vi "Navigation_Main_position_testing april 19.vi"() -> ()   [LabVIEW 2015]
uses:
  <vilib>/myRIO/Common/Instrument Driver Framework/Utilities/typedefs/Generic FPGA Reference.ctl
  <vilib>/myRIO/Common/Instrument Driver Framework/Utilities/typedefs/myRIO v1.0 Reference.ctl
  <vilib>/myRIO/Common/Instrument Driver Framework/Utilities/typedefs/Hardware Version Enum.ctl
  <vilib>/myRIO/Common/Instrument Driver Framework/Utilities/typedefs/myRIO Generic Hardware Reference.ctl
  <vilib>/userdefined/High Color/nirio_resource_hc.ctl
  <vilib>/myRIO/Instrument Drivers/Onboard IO/PWM/typedefs/PWM Configuration.ctl
  <vilib>/myRIO/Instrument Drivers/Onboard IO/PWM/PWM.lvlib
  <vilib>/myRIO/Common/Instrument Driver Framework/myRIO v1.0/PWM/typedefs/PWM Channels Enum.ctl
  <vilib>/myRIO/Instrument Drivers/Onboard IO/PWM/typedefs/PWM Reference.ctl
  <vilib>/myRIO/Instrument Drivers/Onboard IO/PWM/vis/myRIO PWM Open.xnode
  <vilib>/myRIO/Common/Instrument Driver Framework/myRIO v1.0/PWM/vis/myRIO v1.1 Open PWM.vi
  <vilib>/rvi/interface/nirviOpenFPGA/nirviOpenFPGA.xnode
  <vilib>/myRIO/Instrument Drivers/Utilities/Utilities.lvlib
  <vilib>/rvi/interface/nirviReadWriteControl/nirviReadWriteControl.xnode
  NiFpgaLv.dll
  <vilib>/Utility/error.llb/Error Cluster From Error Code.vi
  <vilib>/rvi/interface/Simulation/niFpgaSimulationCallBeginRW.vi
  <vilib>/rvi/errors/niLvFpgaAdjustHostInterfaceError.vi
  Navi/E/FPGA Bitfiles/NavigationProjec_FPGATarget2_FPGAMainNavigati_PWPHW8gwDxI.lvbitx
  <vilib>/addons/control/pid/NI_PID_pid.lvlib
  <vilib>/addons/control/pid/pid.llb/PID (DBL).vi
  <vilib>/FPGAPlugInAG/myRIO-1900/niLvFpga_Open_myRIO-1900.vi
  <vilib>/rvi/interface/common/dynamic/niFpgaDynamicAddResources.vi
panel:
  in  "Boolean":bool=TRUE
  out "stop switch":dbl=1.0
  out "distance to goal":dbl
  out "loc_y":dbl
  out "loc_x":dbl
  out "loc_theta":dbl
  out "start y":dbl
  out "start angle":dbl=1.0
  out "start x":dbl=1.0
  in  "set start position":bool=TRUE
  out "goal reached":bool=TRUE
  out "x/y":dbl
  out "scale":dbl=1.0
  in  "x goal":dbl=10.0
  in  "L Desired Input Velocity (ft/s) 4":dbl(knob) scale=-4.0..4.0
  in  "R Min Linear Velocity (ft/s)  2":dbl=-2.0 format="%#_13g"
  in  "L Min Linear Velocity (ft/s) 9":dbl=-2.0 format="%#_13g"
  in  "R Max Linear Velocity (ft/s) 5":dbl=2.0 format="%#_13g"
  in  "L Max Linear Velocity (ft/s) 5":dbl=2.0 format="%#_13g"
  in  "R Desired Input Velocity (ft/s) 5":dbl(knob) scale=-4.0..4.0
  out "left":dbl
  out "right":dbl
  out "left wheels actual pwm":dbl
  in  "stop 3":bool
  out "left pwm":dbl(graph)
  out "dt out (s) 3":dbl format="%.3f"
  in  "output range 3":cluster{"output high":dbl, "output low":dbl}={"output high"=0.13333, "output low"=-0.13333} {"output low" format="%.6f"; "output high" format="%.5f"}
  in  "PID gains 3":T1={"proportional gain (Kc)"=0.002, "integral time (Ti, min)"=7e-07, "derivative time (Td, min)"=0.0} {"derivative time (Td, min)" format="%.8f"; "integral time (Ti, min)" format="%.8f"; "proportional gain (Kc)" format="%.8f"}
  out "desired pwm 2":dbl
  out "feedback 2":dbl
  out ".not. x? 3":bool
  out "Elapsed Time (s) 2":dbl caption="Elapsed Time (s)"
  out "x traveled 2":dbl
  out "y traveled 2":dbl
  out "avg 124":dbl
  out "avg 457":dbl
  out "psi dot 2":dbl
  out "distance traveled 2":dbl
  out "y dot 2":dbl
  out "x dot 2":dbl
  out "x position 2":dbl
  out "y position 2":dbl
  out "reset x y 2":dbl
  out "Tick Count(mSec) 2":u32 caption="Tick Count(mSec)"
  in  "start y 2":dbl=3.0
  in  "start x 2":dbl=1.0
  out "right wheels actual pwm":dbl
  in  "stop 2":bool
  out "right pwm":dbl(graph)
  out "dt out (s) 2":dbl format="%.3f"
  in  "output range 2":cluster{"output high":dbl, "output low":dbl}={"output high"=0.13333, "output low"=-0.13333} {"output low" format="%.6f"; "output high" format="%.5f"}
  in  "PID gains 2":T1={"proportional gain (Kc)"=0.002, "integral time (Ti, min)"=7e-07, "derivative time (Td, min)"=0.0} {"derivative time (Td, min)" format="%.8f"; "integral time (Ti, min)" format="%.8f"; "proportional gain (Kc)" format="%.8f"}
  out "desired pwm":dbl
  out "feedback":dbl
  out ".not. x? 2":bool
  out "Elapsed Time (s)":dbl
  out "LF Rot Velocity (rot/s)":dbl
  out "LM Rot Velocity (rot/s)":dbl
  out "LR Rot Velocity (rot/s)":dbl
  out "RR Rot Velocity (rot/s)":dbl
  out "RM Linear Velocity (rot/s)":dbl
  out "RF Linear Velocity (rot/s)":dbl
  in  "Encoder Reset":bool
  out "SYS.SELECTA":u8 format="%08b"
  out "ENC.B_c.CNTR":i32
  out "ENC.B_b.CNTR":i32
  out "ENC.B_a.CNTR":i32
  out "ENC.A_c.CNTR":i32
  out "ENC.A_b.CNTR":i32
  out "ENC.A_a.CNTR":i32
  in  "R Min Linear Velocity (ft/s)":dbl=-2.0 format="%#_13g"
  in  "R Max Linear Velocity (ft/s)":dbl=2.0 format="%#_13g"
  in  "L Min Linear Velocity (ft/s)":dbl=-2.0 format="%#_13g"
  in  "L Max Linear Velocity (ft/s)":dbl=2.0 format="%#_13g"
  out "Current Rot Velocity (rot/s)":T2(graph)
  # "Motor Control Parameters"
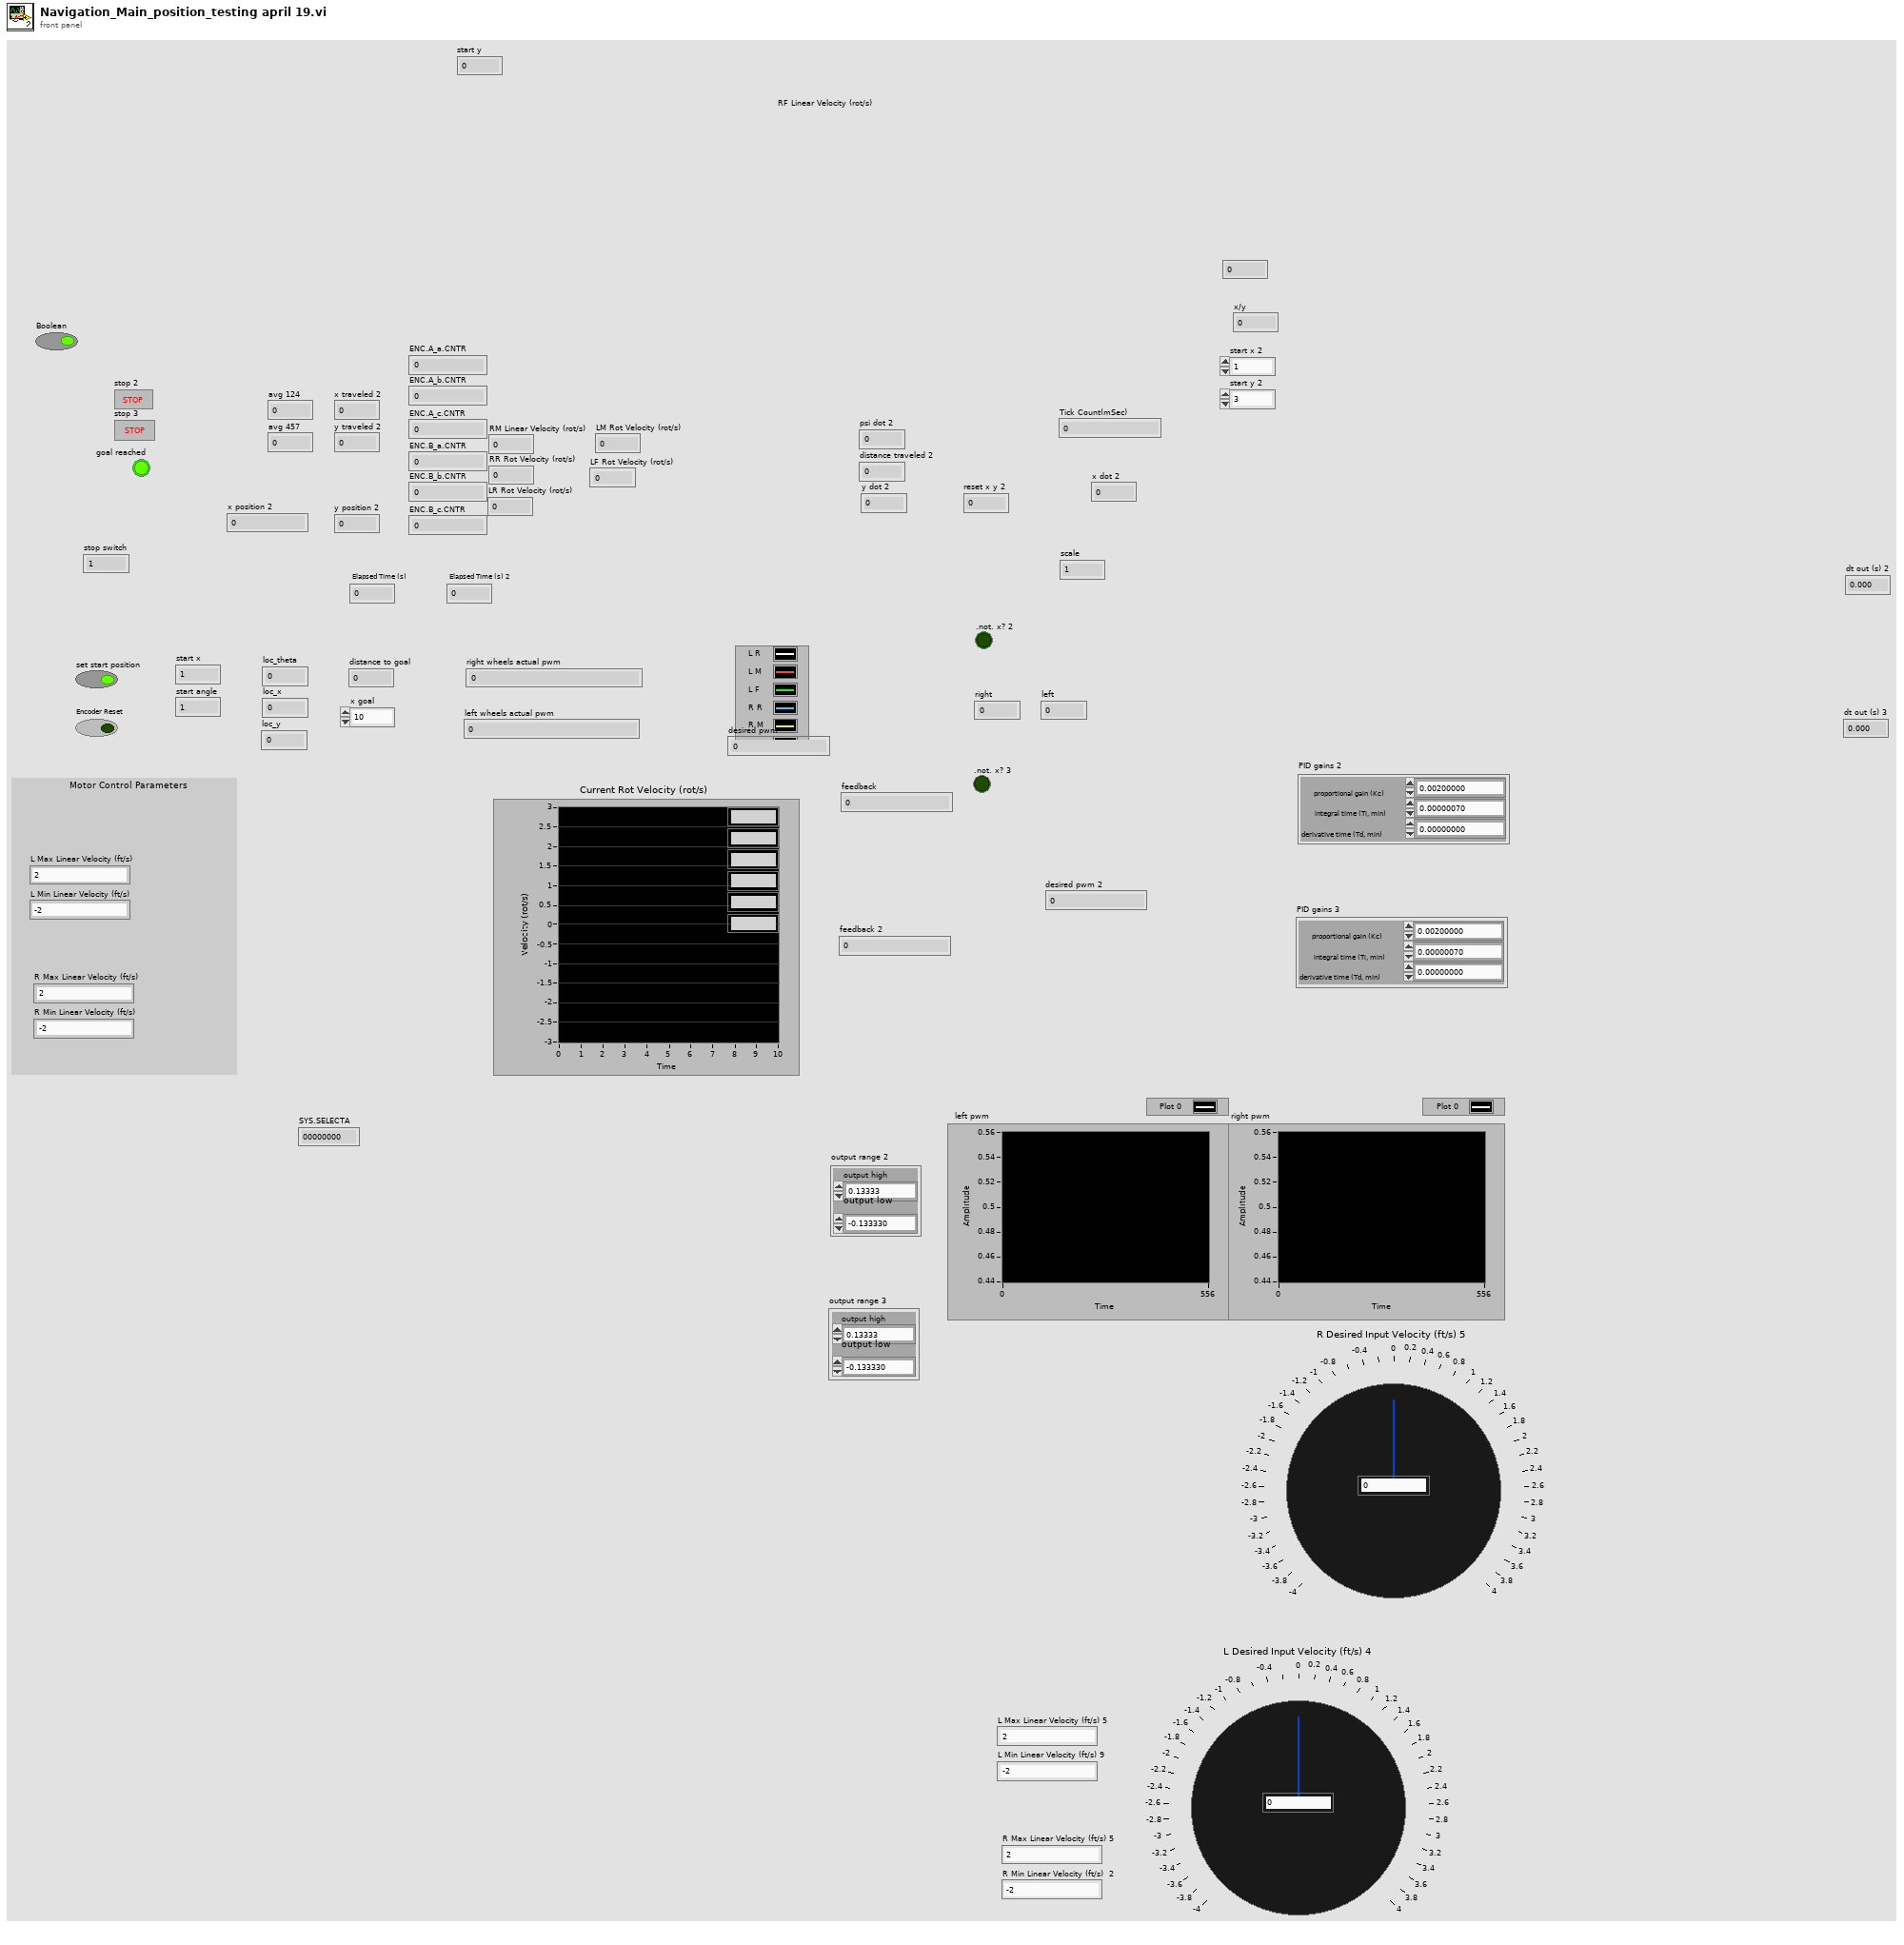
[diagram p1: front panel]
types:
  T1 = cluster{"proportional gain (Kc)":dbl, "integral time (Ti, min)":dbl, "derivative time (Td, min)":dbl}
  T2 = cluster{"Rotational Velocity (RPS)":dbl, "Rotational Velocity (RPS)":dbl, "Rotational Velocity (RPS)":dbl, "Rotational Velocity (RPS)":dbl, "Rotational Velocity (RPS)":dbl, "Rotational Velocity (RPS)":dbl}
  T3 = typedef "nirio_resource_hc.ctl" = tag
  T4 = typedef "Hardware Version Enum.ctl" = enum16{"Unknown", "myRIO-1900", "myRIO-1950", "roboRIO"}
  T5 = typedef "PWM.lvlib/PWM Reference.ctl" = cluster{"myRIO Reference":T6, "PWM Channels Enum":T9, "PWM Configuration":T10}
  T6 = typedef "myRIO Generic Hardware Reference.ctl" = cluster{"myRIO Model":T4, "myRIO Hardware Reference":T7}
  T7 = typedef "myRIO v1.0 Reference.ctl" = cluster{"Generic FPGA Reference":T8, "Allow multiple opens":bool}
  T8 = typedef "Generic FPGA Reference.ctl" = refnum<k20>
  T9 = typedef "PWM Channels Enum.ctl" = enum16{"Not Connected", "C/PWM0", "C/PWM1", "A/PWM0", "A/PWM1", "A/PWM2", "B/PWM0", "B/PWM1", "B/PWM2", "PWM/PWM0", "PWM/PWM1", "PWM/PWM2", "PWM/PWM3", "PWM/PWM4", "PWM/PWM5", "PWM/PWM6", "PWM/PWM7", "PWM/PWM8", "PWM/PWM9"}
  T10 = typedef "PWM.lvlib/PWM Configuration.ctl" = cluster{"Frequency":dbl, "Duty Cycle":dbl}
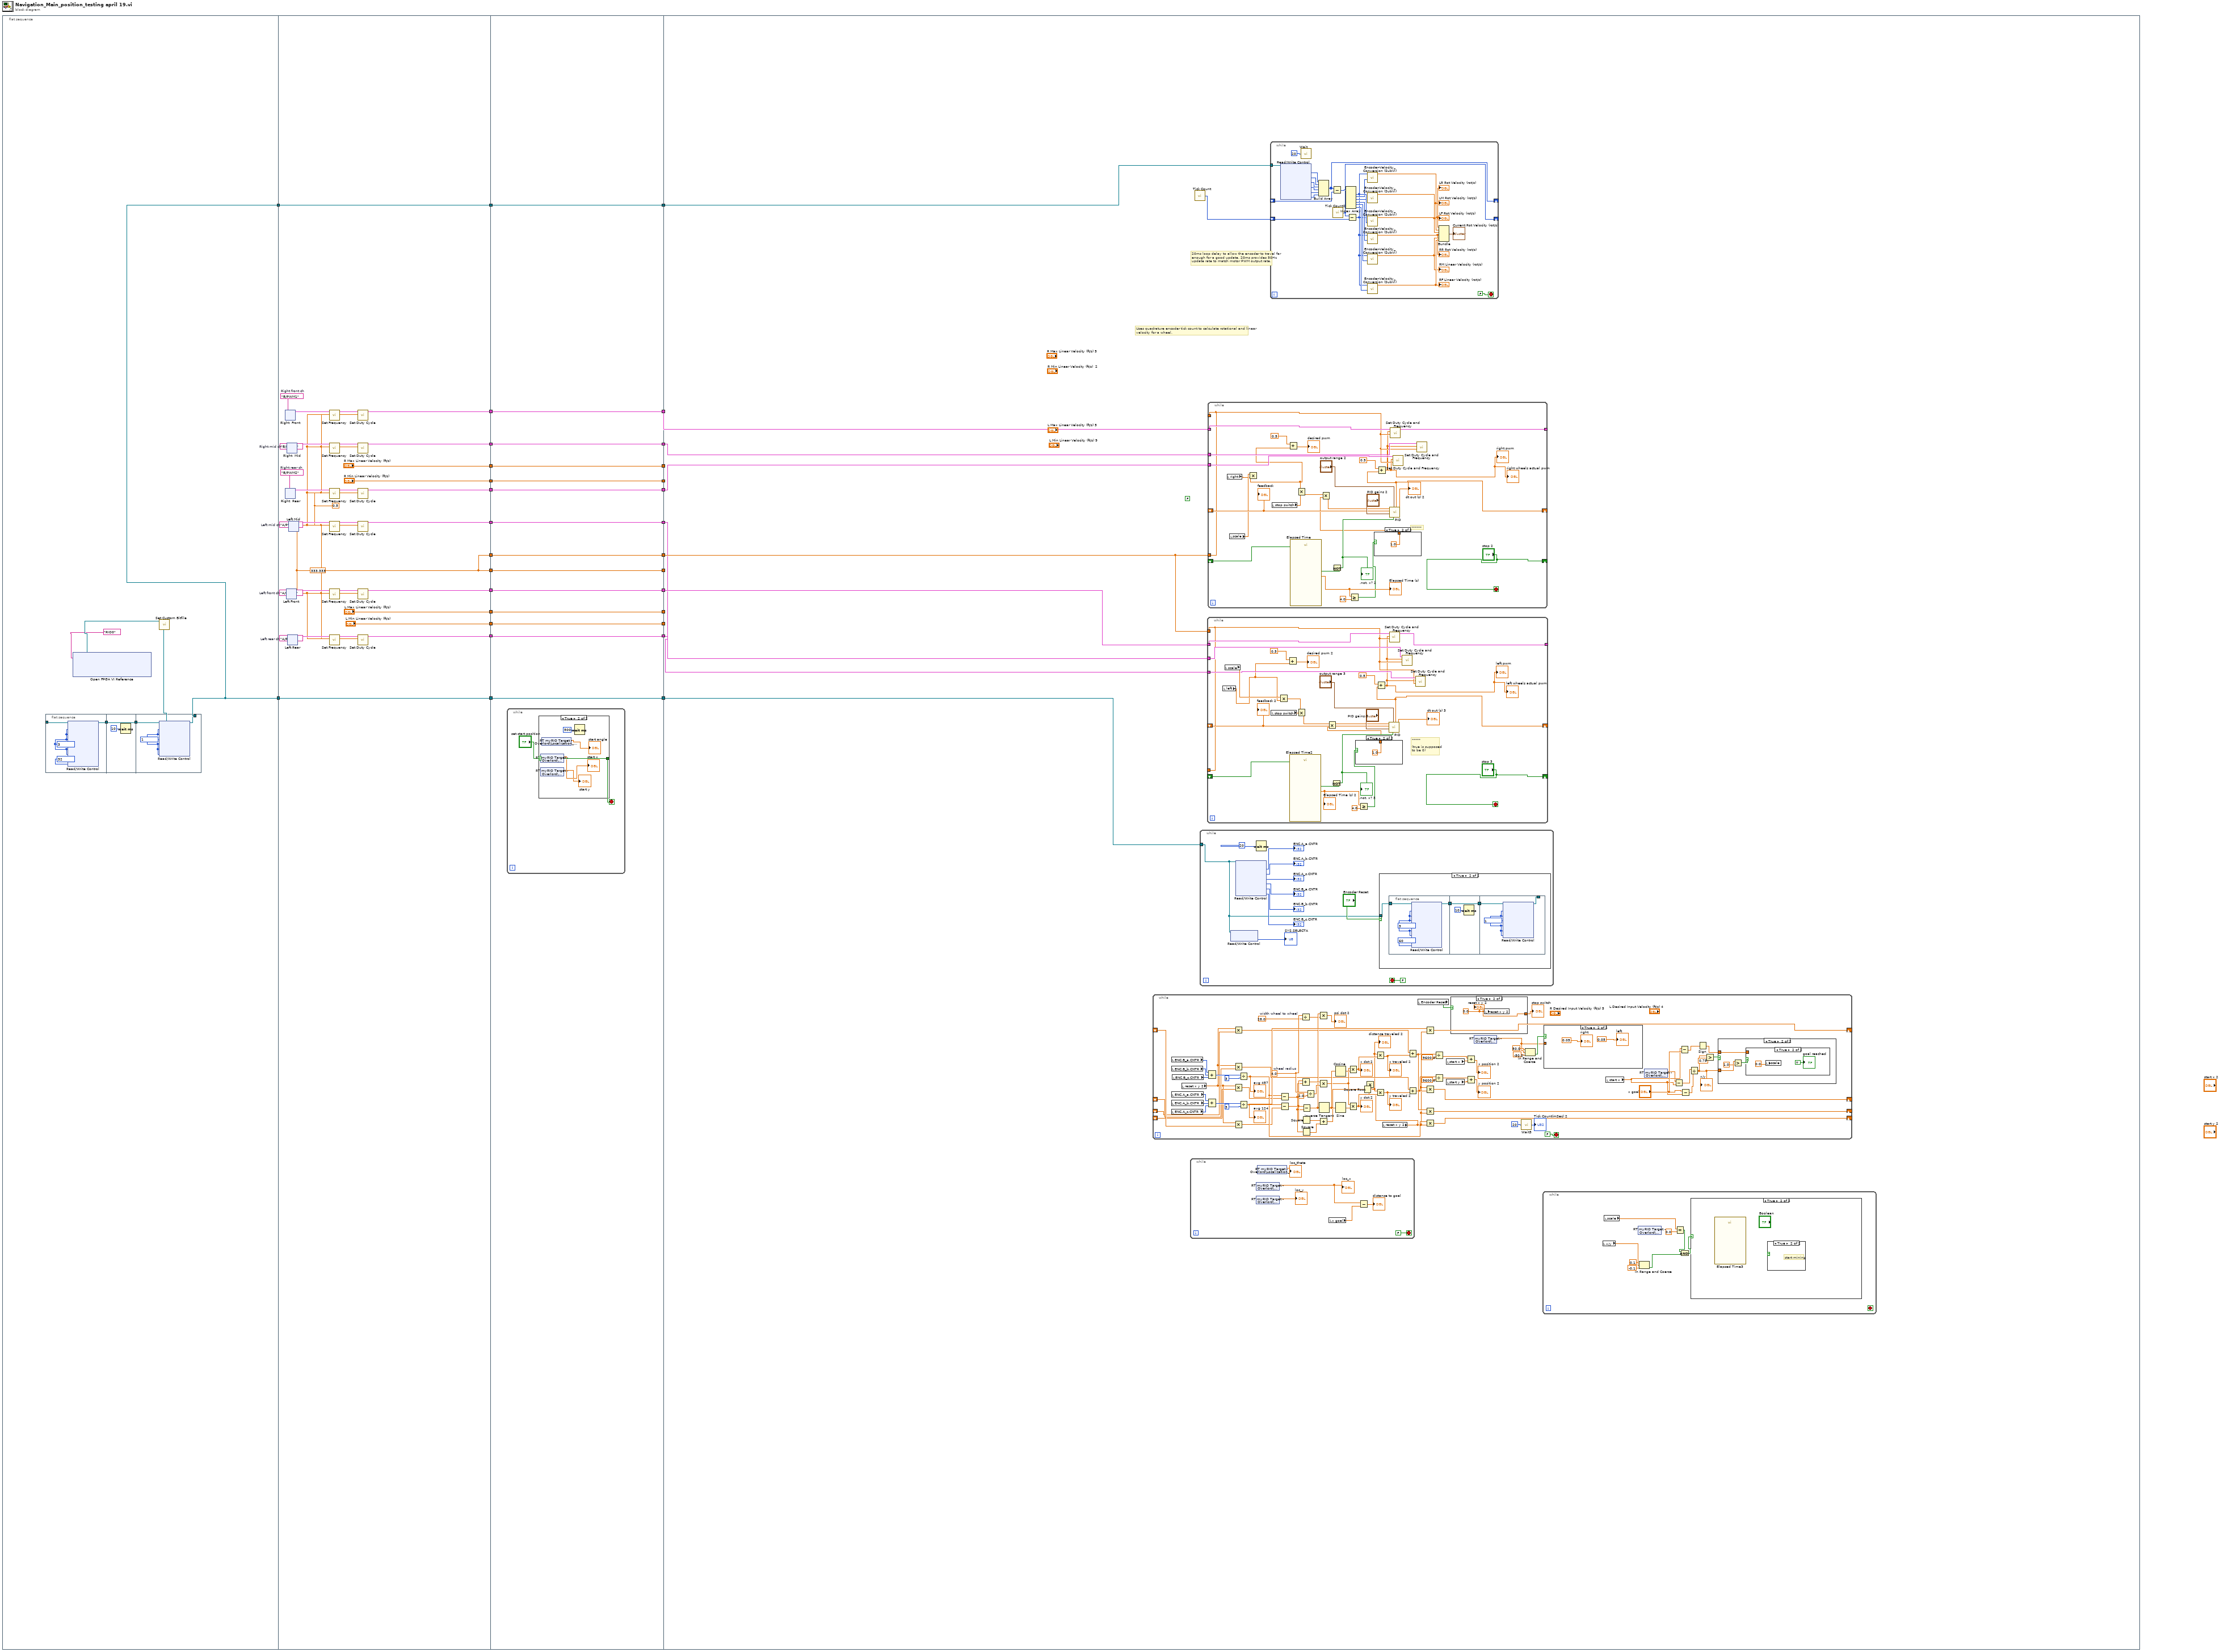
[diagram p0: block diagram]
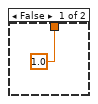
[diagram p5: hidden frame]
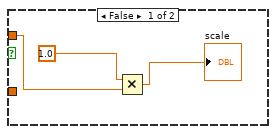
[diagram p6: hidden frame]
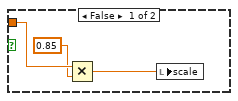
[diagram p7: hidden frame]
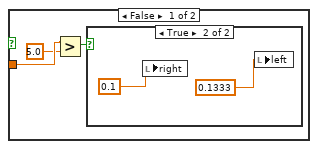
[diagram p8: hidden frame]
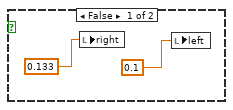
[diagram p9: hidden frame]
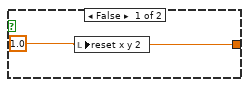
[diagram p10: hidden frame]
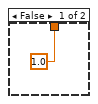
[diagram p11: hidden frame]
diagram:
  n1 = flat-sequence {
    tunnel: [w33] -> w30
    tunnel: [w33] -> w29
    tunnel: [w46] -> w28
    tunnel: [w61] -> w26
    tunnel: [w57] -> w24
    tunnel: [w56] -> w22
    tunnel: [w55] -> w20
    tunnel: [w54] -> w18
    tunnel: [w53] -> w16
    tunnel: ["L Max Linear Velocity (ft/s)"] -> w14
    tunnel: ["L Min Linear Velocity (ft/s)"] -> w12
    tunnel: ["R Max Linear Velocity (ft/s)"] -> w10
    tunnel: ["R Min Linear Velocity (ft/s)"] -> w8
    tunnel: [w48] -> w6
    tunnel: w30 -> [w47]
    tunnel: [w47] -> w4
    tunnel: w29 -> [w48]
    tunnel: [w46] -> w2
    tunnel: w28 -> [w187]
    tunnel: [w187] -> w27
    tunnel: w26 -> [w186]
    tunnel: [w186] -> w25
    tunnel: w24 -> [w185]
    tunnel: [w185] -> w23
    tunnel: w22 -> [w184]
    tunnel: [w184] -> w21
    tunnel: w20 -> [w183]
    tunnel: [w183] -> w19
    tunnel: w18 -> [w182]
    tunnel: [w182] -> w17
    tunnel: w16 -> [w181]
    tunnel: [w181] -> w15
    tunnel: w14 -> [w180]
    tunnel: [w180] -> w13
    tunnel: w12 -> [w179]
    tunnel: [w179] -> w11
    tunnel: w10 -> [w178]
    tunnel: [w178] -> w9
    tunnel: w8 -> [w177]
    tunnel: [w177] -> w7
    tunnel: w6 -> [w176]
    tunnel: [w176] -> w5
    tunnel: w4 -> [w175]
    tunnel: [w175] -> w3
    tunnel: w2 -> [w174]
    tunnel: [w174] -> w1
    tunnel: w27 -> [_]
    tunnel: w25 -> [w195]
    tunnel: w23 -> [w201]
    tunnel: w21 -> [w198]
    tunnel: w19 -> [w197]
    tunnel: w17 -> [w196]
    tunnel: w15 -> [w200]
    tunnel: w13 -> [_]
    tunnel: w11 -> [_]
    tunnel: w9 -> [_]
    tunnel: w7 -> [_]
    tunnel: w5 -> [w203]
    tunnel: w3 -> [w202]
    tunnel: w1 -> [w199]
    frame #0 {
      n2 = flat-sequence {
        tunnel: w34 -> [w39]
        tunnel: [w37] -> w36
        tunnel: w36 -> [w41]
        tunnel: [w41] -> w35
        tunnel: w35 -> [w44]
        tunnel: [w43] -> w33
        frame #0 {
          w38 = u8 32 ("SYS.SELECTA")
          w40 = u8 3 ("ENC.B_c.CNFG")
          n3 = xnode "Read/Write Control"("FPGA VI Reference In"=w39, "ENC.A_a.CNFG"=w40, "ENC.A_b.CNFG"=w40, "ENC.A_c.CNFG"=w40, "ENC.B_a.CNFG"=w40, "ENC.B_b.CNFG"=w40, "ENC.B_c.CNFG"=w40, "SYS.SELECTA"=w38, "SYS.SELECTB"=w38) -> ("FPGA VI Reference Out"=w37:refnum<k20>)  [unwired: 1 in, 1 out]
        }
        frame #1 {
          n4 = Wait (ms)(milliseconds to wait=u32 10) -> ()  [unwired: 1 out]
        }
        frame #2 {
          w45 = u8 1 ("ENC.B_c.CNFG")
          n5 = xnode "Read/Write Control"("FPGA VI Reference In"=w44, "ENC.A_a.CNFG"=w45, "ENC.A_b.CNFG"=w45, "ENC.A_c.CNFG"=w45, "ENC.B_a.CNFG"=w45, "ENC.B_b.CNFG"=w45, "ENC.B_c.CNFG"=w45) -> ("FPGA VI Reference Out"=w43:refnum<k20>)  [unwired: 1 in, 1 out]
        }
      }
      n6 = xnode "Open FPGA VI Reference"("resource name"=tag "RIO0") -> ("FPGA VI Reference Out"=w32:refnum<k20>)  [unwired: 1 in, 1 out]
      n7 = call <vilib>:"Set Custom Bitfile.vi"("Custom FPGA Reference In"=w32) -> ("Custom FPGA Reference Out"=w34:refnum<k20>)  [unwired: 9 in, 1 out]
    }
    frame #1 {
      w58 = 0.5 ("Duty Cycle")
      w46 = 333.333 ("Frequency [Hz]")
      w72 = tag "B/PWM2"  # Right rear ch
      w73 = tag "B/PWM0"  # Right mid ch
      w74 = tag "B/PWM1"  # Right front ch
      w75 = tag "A/PWM2"  # Left rear ch
      w76 = tag "A/PWM1"  # Left mid ch
      w77 = tag "A/PWM0"  # Left front ch
      n8 = xnode "Right  Front"("Channel Name"=w74) -> ("PWM Ref Out"=w68:T5)  [unwired: 2 in, 1 out]
      n9 = xnode "Right  Rear"("Channel Name"=w72) -> ("PWM Ref Out"=w66:T5)  [unwired: 2 in, 1 out]
      n10 = xnode "Left Front"("Channel Name"=w77) -> ("PWM Ref Out"=w71:T5)  [unwired: 2 in, 1 out]
      n11 = xnode "Right  Mid"("Channel Name"=w73) -> ("PWM Ref Out"=w67:T5)  [unwired: 2 in, 1 out]
      n12 = xnode "Left Rear"("Channel Name"=w75) -> ("PWM Ref Out"=w69:T5)  [unwired: 2 in, 1 out]
      n13 = xnode "Left Mid"("Channel Name"=w76) -> ("PWM Ref Out"=w70:T5)  [unwired: 2 in, 1 out]
      n14 = call <vilib>:"Set Frequency.vi"("Frequency [Hz]"=w46, "PWM Ref In"=w68) -> ("PWM Ref Out"=w62:T5)  [unwired: 7 in, 1 out]
      n15 = call <vilib>:"Set Frequency.vi"("Frequency [Hz]"=w46, "PWM Ref In"=w67) -> ("PWM Ref Out"=w63:T5)  [unwired: 7 in, 1 out]
      n16 = call <vilib>:"Set Frequency.vi"("Frequency [Hz]"=w46, "PWM Ref In"=w66) -> ("PWM Ref Out"=w64:T5)  [unwired: 7 in, 1 out]
      n17 = call <vilib>:"Set Frequency.vi"("Frequency [Hz]"=w46, "PWM Ref In"=w70) -> ("PWM Ref Out"=w59:T5)  [unwired: 7 in, 1 out]
      n18 = call <vilib>:"Set Frequency.vi"("Frequency [Hz]"=w46, "PWM Ref In"=w71) -> ("PWM Ref Out"=w65:T5)  [unwired: 7 in, 1 out]
      n19 = call <vilib>:"Set Frequency.vi"("Frequency [Hz]"=w46, "PWM Ref In"=w69) -> ("PWM Ref Out"=w60:T5)  [unwired: 7 in, 1 out]
      n20 = call <vilib>:"Set Duty Cycle.vi"("Duty Cycle"=w58, "PWM Ref In"=w62) -> ("PWM Ref Out"=w57:T5)  [unwired: 7 in, 1 out]
      n21 = call <vilib>:"Set Duty Cycle.vi"("Duty Cycle"=w58, "PWM Ref In"=w63) -> ("PWM Ref Out"=w56:T5)  [unwired: 7 in, 1 out]
      n22 = call <vilib>:"Set Duty Cycle.vi"("Duty Cycle"=w58, "PWM Ref In"=w64) -> ("PWM Ref Out"=w55:T5)  [unwired: 7 in, 1 out]
      n23 = call <vilib>:"Set Duty Cycle.vi"("Duty Cycle"=w58, "PWM Ref In"=w59) -> ("PWM Ref Out"=w54:T5)  [unwired: 7 in, 1 out]
      n24 = call <vilib>:"Set Duty Cycle.vi"("Duty Cycle"=w58, "PWM Ref In"=w65) -> ("PWM Ref Out"=w53:T5)  [unwired: 7 in, 1 out]
      n25 = call <vilib>:"Set Duty Cycle.vi"("Duty Cycle"=w58, "PWM Ref In"=w60) -> ("PWM Ref Out"=w61:T5)  [unwired: 7 in, 1 out]
    }
    frame #2 {
      n26 = while {
        stop <- w188 stop-if-true
        n27 = case shown="True" "set start position" {
          selector: "set start position" -> [_ w194]
          tunnel: [_ w194] -> w188
          frame False {
          }
          frame True {
            n28 = shared-variable "RT myRIO Target - Overlord\\Localization_Variables_r0.lvlib\\loc_x"() -> (→"start x":dbl)  [unwired: 1 in, 1 out]
            n29 = shared-variable "RT myRIO Target - Overlord\\Localization_Variables_r0.lvlib\\loc_y"() -> (→"start y":dbl)  [unwired: 1 in, 1 out]
            n30 = shared-variable "RT myRIO Target - Overlord\\Localization_Variables_r0.lvlib\\loc_theta"() -> (→"start angle":dbl)  [unwired: 1 in, 1 out]
            n31 = Wait (ms)(milliseconds to wait=u32 500) -> ()  [unwired: 1 out]
          }
        }
      }
    }
    frame #3 {
      (unwired) FALSE
      # "Uses quadrature encoder tick count to calculate rotational and linear velocity for a wheel."
      # "20ms loop delay to allow the encoder to travel far enough for a good update. 20ms provides 50Hz update rate to match motor PWM output rate."
      n32 = while {
        shift-right: [w275] -> _
        shift-left: _ -> [w313]
        shift-right: [w272] -> _
        shift-left: _ -> [w312]
        shift-right: [w274] -> _
        shift-left: _ -> [w287]
        shift-right: [w273] -> _
        shift-left: _ -> [w286]
        stop <- FALSE stop-if-true
        w308 = 28.0  # width wheel to wheel
        w309 = 4.0  # wheel radius
        n33 = local read "ENC.B_a.CNTR"() -> (w318:i32)
        n34 = local read "ENC.B_b.CNTR"() -> (w317:i32)
        n35 = local read "ENC.A_a.CNTR"() -> (w321:i32)
        n36 = local read "ENC.A_b.CNTR"() -> (w320:i32)
        n37 = local read "ENC.A_c.CNTR"() -> (w319:i32)
        n38 = local read "ENC.B_c.CNTR"() -> (w316:i32)
        n39 = local read "reset x y 2"() -> (w271:dbl)
        n40 = Compound Arithmetic op=ADD(w318, w317, w316) -> (w324:i32)
        n41 = Compound Arithmetic op=ADD(w321, w320, w319) -> (w325:i32)
        n42 = Multiply(x=w271, y=w286) -> (x*y=w277:dbl)
        n43 = Multiply(x=w271, y=w287) -> (x*y=w278:dbl)
        n44 = Multiply(x=w271, y=w312) -> (x*y=w276:dbl)
        n45 = Multiply(x=w271, y=w313) -> (x*y=w279:dbl)
        n46 = Divide(x=w324, y=3) -> (x/y=w311:dbl)
        "avg 457" <- w311
        n47 = Divide(x=w325, y=3) -> (x/y=w314:dbl)
        "avg 124" <- w314
        n48 = Subtract(x=w311, y=w276) -> (x-y=w301:dbl)
        n49 = Subtract(x=w314, y=w279) -> (x-y=w302:dbl)
        n50 = Divide(x=w309, y=w308) -> (x/y=w304:dbl)
        n51 = Add(x=w302, y=w301) -> (x+y=w306:dbl)
        n52 = Square(x=w302) -> (x^2=w299:dbl)
        n53 = Square(x=w301) -> (x^2=w300:dbl)
        n54 = Subtract(x=w302, y=w301) -> (x-y=w305:dbl)
        n55 = Divide(x=w309, y=2.0) -> (x/y=w307:dbl)
        n56 = Multiply(x=w305, y=w304) -> (x*y=→"psi dot 2":dbl)
        n57 = Multiply(x=w306, y=w307) -> (x*y=w295:dbl)
        n58 = Add(x=w299, y=w300) -> (x+y=w298:dbl)
        n59 = Inverse Tangent(1:w305) -> (0:w303:dbl)
        n60 = Cosine(x=w303) -> (cos(x)=w296:dbl)
        n61 = Sine(x=w303) -> (sin(x)=w297:dbl)
        n62 = Multiply(x=w295, y=w296) -> (x*y=w293:dbl)
        "x dot 2" <- w293
        n63 = Multiply(x=w295, y=w297) -> (x*y=w294:dbl)
        "y dot 2" <- w294
        n64 = Square Root(x=w298) -> (sqrt(x)=w292:dbl)
        n65 = local read "reset x y 2"() -> (w269:dbl)
        n66 = Multiply(x=w292, y=w269) -> (x*y=w270:dbl)
        "distance traveled 2" <- w270
        n67 = Multiply(x=w270, y=w293) -> (x*y=w291:dbl)
        "x traveled 2" <- w291
        n68 = Multiply(x=w270, y=w294) -> (x*y=w290:dbl)
        "y traveled 2" <- w290
        n69 = Add(x=w277, y=w291) -> (x+y=w289:dbl)
        n70 = Add(x=w278, y=w290) -> (x+y=w281:dbl)
        n71 = local read "Encoder Reset"() -> (w268:bool)
        n72 = Multiply(x=w314, y=w269) -> (x*y=w275:dbl)
        n73 = Multiply(x=w269, y=w281) -> (x*y=w274:dbl)
        n74 = Multiply(x=w289, y=w269) -> (x*y=w273:dbl)
        n75 = Multiply(x=w311, y=w269) -> (x*y=w272:dbl)
        n76 = Divide(x=w289, y=9600.0) -> (x/y=w284:dbl)
        n77 = Divide(x=w281, y=9600.0) -> (x/y=w285:dbl)
        n78 = local read "start x"() -> (w282:dbl)
        n79 = local read "start y"() -> (w283:dbl)
        n80 = case shown="True" w268 {
          tunnel: [w348 w349] -> w249
          frame False {
            w348 = 1.0
            n81 = local write "reset x y 2"(w348) -> ()
          }
          frame True {
            w349 = 0.0
            n82 = local write "reset x y 2"(w349) -> ()
            "reset x y 2" <- w349
          }
        }
        "stop switch" <- w249
        n83 = Add(x=w284, y=w282) -> (x+y=→"x position 2":dbl)
        n84 = Add(x=w285, y=w283) -> (x+y=→"y position 2":dbl)
        n85 = shared-variable "RT myRIO Target - Overlord\\Localization_Variables_r0.lvlib\\loc_x"() -> (w251:dbl)  [unwired: 1 in, 1 out]
        n86 = call "Wait3"("Count(mSec)"=u32 20) -> ("Tick Count(mSec)"=→"Tick Count(mSec) 2":u32)
        n87 = In Range and Coerce(upper limit=50.0, x=w251, lower limit=-50.0) -> (In Range?=w262:bool)  [unwired: 1 out]
        n88 = case shown="True" w262 {
          tunnel: w251 -> [w341 _]
          frame False {
            n89 = Greater?(x=w341, y=5.0) -> (0:w339:bool)
            n90 = case shown="True" w339 {
              frame False {
                n91 = local write "right"(0.133) -> ()
                n92 = local write "left"(0.1) -> ()
              }
              frame True {
                n93 = local write "right"(0.1) -> ()
                n94 = local write "left"(0.1333) -> ()
              }
            }
          }
          frame True {
            "right" <- 0.05
            "left" <- 0.05
          }
        }
        n95 = local read "start x"() -> (w253:dbl)
        n96 = shared-variable "RT myRIO Target - Overlord\\Localization_Variables_r0.lvlib\\loc_x"() -> (w250:dbl)  [unwired: 1 in, 1 out]
        n97 = Subtract(x=w250, y=w253) -> (x-y=w258:dbl)
        n98 = Subtract(x=w253, y="x goal") -> (x-y=w255:dbl)
        n99 = Subtract(x="x goal", y=w253) -> (x-y=w257:dbl)
        n100 = Divide(x=w258, y=w257) -> (x/y=w259:dbl)
        "x/y" <- w259
        n101 = Sign(1:w255) -> (0:w254:dbl)
        n102 = Greater?(x=w259, y=0.75) -> (0:w260:bool)
        n103 = case shown="True" w260 {
          tunnel: w259 -> [_ w333]
          tunnel: w254 -> [w328 w330]
          frame False {
            n104 = Multiply(x=1.0, y=w328) -> (x*y=→"scale":dbl)
          }
          frame True {
            n105 = Greater?(x=w333, y=1.0) -> (0:w331:bool)
            n106 = case shown="True" w331 {
              tunnel: w330 -> [w336 _]
              frame False {
                n107 = Multiply(x=w336, y=0.85) -> (x*y=w334:dbl)
                n108 = local write "scale"(w334) -> ()
              }
              frame True {
                n109 = local write "scale"(0.0) -> ()
                "goal reached" <- TRUE
              }
            }
          }
        }
      }
      n110 = while {
        stop <- FALSE stop-if-true
        n111 = shared-variable "RT myRIO Target - Overlord\\Localization_Variables_r0.lvlib\\loc_x"() -> (w216:dbl)  [unwired: 1 in, 1 out]
        "loc_x" <- w216
        n112 = shared-variable "RT myRIO Target - Overlord\\Localization_Variables_r0.lvlib\\loc_y"() -> (→"loc_y":dbl)  [unwired: 1 in, 1 out]
        n113 = shared-variable "RT myRIO Target - Overlord\\Localization_Variables_r0.lvlib\\loc_theta"() -> (→"loc_theta":dbl)  [unwired: 1 in, 1 out]
        n114 = local read "x goal"() -> (w215:dbl)
        n115 = Subtract(x=w216, y=w215) -> (x-y=→"distance to goal":dbl)
      }
      n116 = call "Tick Count"() -> ("Tick Count(uSec)"=w204:u32)
      n117 = while {
        tunnel: w203 -> [w380]
        stop <- FALSE stop-if-true
        n118 = xnode "Read/Write Control"("FPGA VI Reference In"=w380) -> ("SYS.SELECTA"=→"SYS.SELECTA":u8)  [unwired: 1 in, 2 out]
        n119 = xnode "Read/Write Control"("FPGA VI Reference In"=w380) -> ("ENC.A_a.CNTR"=→"ENC.A_a.CNTR":u32, "ENC.A_b.CNTR"=→"ENC.A_b.CNTR":u32, "ENC.A_c.CNTR"=→"ENC.A_c.CNTR":u32, "ENC.B_a.CNTR"=→"ENC.B_a.CNTR":u32, "ENC.B_b.CNTR"=→"ENC.B_b.CNTR":u32, "ENC.B_c.CNTR"=→"ENC.B_c.CNTR":u32)  [unwired: 1 in, 2 out]
        n120 = Wait (ms)(milliseconds to wait=u32 20) -> ()  [unwired: 1 out]
        n121 = case shown="True" "Encoder Reset" {
          tunnel: w380 -> [_ w391]
          frame False {
          }
          frame True {
            n122 = flat-sequence {
              tunnel: w391 -> [w396]
              tunnel: [w394] -> w393
              tunnel: w393 -> [w398]
              tunnel: [w398] -> w392
              tunnel: w392 -> [w401]
              tunnel: [w400] -> _
              frame #0 {
                w395 = u8 60 ("SYS.SELECTA")
                w397 = u8 3 ("ENC.B_c.CNFG")
                n123 = xnode "Read/Write Control"("FPGA VI Reference In"=w396, "ENC.A_a.CNFG"=w397, "ENC.A_b.CNFG"=w397, "ENC.A_c.CNFG"=w397, "ENC.B_a.CNFG"=w397, "ENC.B_b.CNFG"=w397, "ENC.B_c.CNFG"=w397, "SYS.SELECTA"=w395, "SYS.SELECTB"=w395) -> ("FPGA VI Reference Out"=w394:refnum<k20>)  [unwired: 1 in, 1 out]
              }
              frame #1 {
                n124 = Wait (ms)(milliseconds to wait=u32 10) -> ()  [unwired: 1 out]
              }
              frame #2 {
                w402 = u8 1 ("ENC.B_c.CNFG")
                n125 = xnode "Read/Write Control"("FPGA VI Reference In"=w401, "ENC.A_a.CNFG"=w402, "ENC.A_b.CNFG"=w402, "ENC.A_c.CNFG"=w402, "ENC.B_a.CNFG"=w402, "ENC.B_b.CNFG"=w402, "ENC.B_c.CNFG"=w402) -> ("FPGA VI Reference Out"=w400:refnum<k20>)  [unwired: 1 in, 1 out]
              }
            }
          }
        }
      }
      n126 = while {
        tunnel: w200 -> [w245]
        tunnel: [w246] -> _
        tunnel: w199 -> [w232]
        shift-right: [w231] -> _
        shift-left: _ -> [w241]
        shift-right: ["stop 3"] -> _
        shift-left: _ -> [w223]
        tunnel: [w232] -> _
        tunnel: w196 -> [w234]
        tunnel: w195 -> [w233]
        stop <- "stop 3" stop-if-true
        # "*****\n\n(true is supposed\nto be 0)"
        n127 = local read "left"() -> (w230:dbl)
        n128 = local read "scale"() -> (w235:dbl)
        n129 = local read "stop switch"() -> (w227:dbl)
        n130 = Multiply(x=w235, y=w230) -> (x*y=w229:dbl)
        n131 = Add(x=0.5, y=w230) -> (x+y=→"desired pwm 2":dbl)
        n132 = call "Elapsed Time2"("Reset"=w223) -> ("Elapsed Time (s)"=w222:dbl, "Time has Elapsed"=w226:bool)  [unwired: 11 in, 6 out]
        "Elapsed Time (s) 2" <- w222
        n133 = Multiply(x=w229, y=w227) -> (x*y=w228:dbl)
        n134 = Not(x=w226) -> (.not. x?=w239:bool)
        ".not. x? 3" <- w239
        n135 = Greater Or Equal?(x=w222, y=4.0) -> (x >= y?=w220:bool)
        n136 = case shown="True" w220 {
          tunnel: [1.0 1.0] -> w224
          frame False {
          }
          frame True {
          }
        }
        n137 = Multiply(x=w228, y=w224) -> (x*y=w225:dbl)
        n138 = call-poly <vilib>:"PID.vi"("reinitialize? (F)"=w239, "output range"="output range 3", "PID gains"="PID gains 3", "process variable"=w241, "setpoint"=w225) -> ("dt out (s)"=→"dt out (s) 3":dbl, "output"=w231:dbl)  [unwired: 5 in]
        n139 = Add(x=0.5, y=w231) -> (x+y=w219:dbl)
        "left wheels actual pwm" <- w219
        "left pwm" <- w219
        n140 = call <vilib>:"Set Duty Cycle and Frequency.vi"("Frequency [Hz]"=w232, "Duty Cycle"=w219, "PWM Ref In"=w245) -> ("PWM Ref Out"=w246:T5)  [unwired: 6 in, 1 out]
        n141 = call <vilib>:"Set Duty Cycle and Frequency.vi"("Frequency [Hz]"=w232, "Duty Cycle"=w219, "PWM Ref In"=w234) -> ()  [unwired: 6 in, 2 out]
        n142 = call <vilib>:"Set Duty Cycle and Frequency.vi"("Frequency [Hz]"=w232, "Duty Cycle"=w219, "PWM Ref In"=w233) -> ()  [unwired: 6 in, 2 out]
        "feedback 2" <- w241
      }
      n143 = while {
        tunnel: w201 -> [w376]
        tunnel: [w377] -> _
        tunnel: [w363] -> _
        shift-right: [w362] -> _
        shift-left: _ -> [w372]
        shift-right: ["stop 2"] -> _
        shift-left: _ -> [w355]
        tunnel: w199 -> [w363]
        tunnel: w198 -> [w365]
        tunnel: w197 -> [w364]
        stop <- "stop 2" stop-if-true
        # "******"
        n144 = local read "right"() -> (w361:dbl)
        n145 = local read "scale"() -> (w366:dbl)
        n146 = Multiply(x=w366, y=w361) -> (x*y=w360:dbl)
        n147 = local read "stop switch"() -> (w358:dbl)
        n148 = Add(x=0.5, y=w360) -> (x+y=→"desired pwm":dbl)
        n149 = call "Elapsed Time"("Reset"=w355) -> ("Elapsed Time (s)"=w354:dbl, "Time has Elapsed"=w352:bool)  [unwired: 11 in, 6 out]
        "Elapsed Time (s)" <- w354
        n150 = Multiply(x=w360, y=w358) -> (x*y=w359:dbl)
        n151 = Not(x=w352) -> (.not. x?=w370:bool)
        ".not. x? 2" <- w370
        n152 = Greater Or Equal?(x=w354, y=4.0) -> (x >= y?=w351:bool)
        n153 = case shown="True" w351 {
          tunnel: [1.0 1.0] -> w356
          frame False {
          }
          frame True {
          }
        }
        n154 = Multiply(x=w359, y=w356) -> (x*y=w357:dbl)
        n155 = call-poly <vilib>:"PID.vi"("reinitialize? (F)"=w370, "output range"="output range 2", "PID gains"="PID gains 2", "process variable"=w372, "setpoint"=w357) -> ("dt out (s)"=→"dt out (s) 2":dbl, "output"=w362:dbl)  [unwired: 5 in]
        n156 = Add(x=0.5, y=w362) -> (x+y=w350:dbl)
        "right wheels actual pwm" <- w350
        "right pwm" <- w350
        n157 = call <vilib>:"Set Duty Cycle and Frequency.vi"("Frequency [Hz]"=w363, "Duty Cycle"=w350, "PWM Ref In"=w376) -> ("PWM Ref Out"=w377:T5)  [unwired: 6 in, 1 out]
        n158 = call <vilib>:"Set Duty Cycle and Frequency.vi"("Frequency [Hz]"=w363, "Duty Cycle"=w350, "PWM Ref In"=w364) -> ()  [unwired: 6 in, 2 out]
        n159 = call <vilib>:"Set Duty Cycle and Frequency.vi"("Frequency [Hz]"=w363, "Duty Cycle"=w350, "PWM Ref In"=w365) -> ()  [unwired: 6 in, 2 out]
        "feedback" <- w372
      }
      n160 = while {
        shift-right: [w421] -> _
        shift-left: _ -> [w420]
        shift-right: [w418] -> _
        shift-left: w204 -> [w417]
        tunnel: w202 -> [w428]
        stop <- FALSE stop-if-true
        n161 = xnode "Read/Write Control"("FPGA VI Reference In"=w428) -> ("ENC.A_a.CNTR"=w427:u32, "ENC.A_b.CNTR"=w426:u32, "ENC.A_c.CNTR"=w425:u32, "ENC.B_a.CNTR"=w424:u32, "ENC.B_b.CNTR"=w423:u32, "ENC.B_c.CNTR"=w422:u32)  [unwired: 1 in, 2 out]
        n162 = call "Wait"("Count(mSec)"=u32 20) -> ()  [unwired: 1 out]
        n163 = Build Array(w427, w426, w425, w424, w423, w422) -> (w421:u32[])
        n164 = Subtract(x=w421, y=w420) -> (x-y=w419:u32[])
        n165 = call "Tick Count2"() -> ("Tick Count(uSec)"=w418:u32)
        n166 = Index Array(array=w419) -> (element #1=w416:u32, element #2=w415:u32, element #3=w414:u32, element #4=w413:u32, element #5=w412:u32, element #6=w411:u32)  [unwired: 6 in]
        n167 = Subtract(x=w418, y=w417) -> (x-y=w410:u32)
        n168 = call "Encoder-Velocity_Conversion (SubVI).vi"("delta  Encoder Count"=w415, "dt (uSec)"=w410) -> ("Rotational Velocity (RPS)"=w405:dbl)  [unwired: 7 in, 2 out]
        "LM Rot Velocity (rot/s)" <- w405
        n169 = call "Encoder-Velocity_Conversion (SubVI).vi"("delta  Encoder Count"=w414, "dt (uSec)"=w410) -> ("Rotational Velocity (RPS)"=w404:dbl)  [unwired: 7 in, 2 out]
        "LF Rot Velocity (rot/s)" <- w404
        n170 = call "Encoder-Velocity_Conversion (SubVI).vi"("delta  Encoder Count"=w416, "dt (uSec)"=w410) -> ("Rotational Velocity (RPS)"=w406:dbl)  [unwired: 7 in, 2 out]
        "LR Rot Velocity (rot/s)" <- w406
        n171 = call "Encoder-Velocity_Conversion (SubVI).vi"("delta  Encoder Count"=w413, "dt (uSec)"=w410) -> ("Rotational Velocity (RPS)"=w403:dbl)  [unwired: 7 in, 2 out]
        "RR Rot Velocity (rot/s)" <- w403
        n172 = call "Encoder-Velocity_Conversion (SubVI).vi"("delta  Encoder Count"=w412, "dt (uSec)"=w410) -> ("Rotational Velocity (RPS)"=w407:dbl)  [unwired: 7 in, 2 out]
        "RM Linear Velocity (rot/s)" <- w407
        n173 = call "Encoder-Velocity_Conversion (SubVI).vi"("delta  Encoder Count"=w411, "dt (uSec)"=w410) -> ("Rotational Velocity (RPS)"=w408:dbl)  [unwired: 7 in, 2 out]
        "RF Linear Velocity (rot/s)" <- w408
        n174 = Bundle("Rotational Velocity (RPS)"=w406, "Rotational Velocity (RPS)"=w405, "Rotational Velocity (RPS)"=w404, "Rotational Velocity (RPS)"=w403, "Rotational Velocity (RPS)"=w407, "Rotational Velocity (RPS)"=w408) -> (→"Current Rot Velocity (rot/s)":T2)  [unwired: 1 in]
      }
      n175 = while {
        stop <- _ stop-if-true
        n176 = local read "x/y"() -> (w208:dbl)
        n177 = local read "scale"() -> (w211:dbl)
        n178 = shared-variable "RT myRIO Target - Overlord\\Localization_Variables_r0.lvlib\\loc_x"() -> ()  [unwired: 1 in, 2 out]
        n179 = In Range and Coerce(upper limit=0.1, x=w208, lower limit=-0.1) -> (In Range?=w205:bool)  [unwired: 1 out]
        n180 = Equal?(x=w211, y=0.0) -> (x = y?=w210:bool)
        n181 = And(x=w210, y=w205) -> (x .and. y?=w209:bool)
        n182 = case shown="True" w209 {
          frame False {
          }
          frame True {
            n183 = call "Elapsed Time3"() -> ()  [unwired: 12 in, 8 out]
            n184 = case shown="True" {
              selector: _ -> [_ _]
              frame False {
              }
              frame True {
                # "start mining"
              }
            }
          }
        }
      }
    }
  }
